vi "DOE Dryer NI Data Compile.vi"(4 "Module Data 6":string[][](array[string]), 5 "Module Data 7":string[][](array[string]), 6 "Module Data 5":string[][](array[string]), 7 "Module Data 1":string[][](array[string]), 8 "Error In":errorcluster, 9 "Module Data 4":string[][](array[string]), 10 "Module Data 3":string[][](array[string]), 11 "Module Data 2":string[][](array[string])) -> (0 "Error Out":errorcluster, 3 "Data Output":string[][](array[string]))   [LabVIEW 2018]
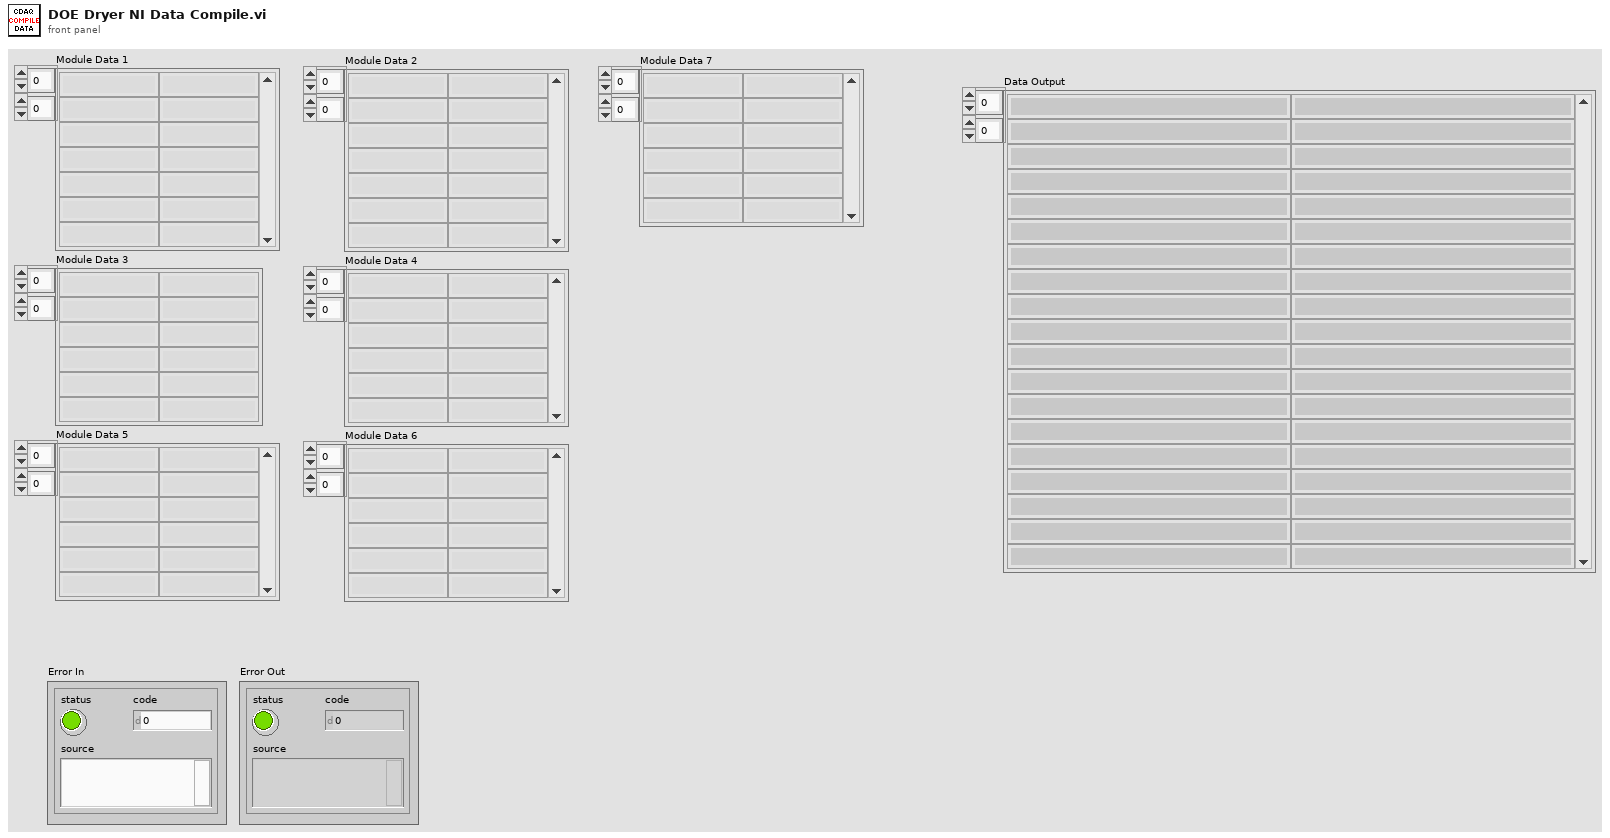
[diagram p1: front panel]
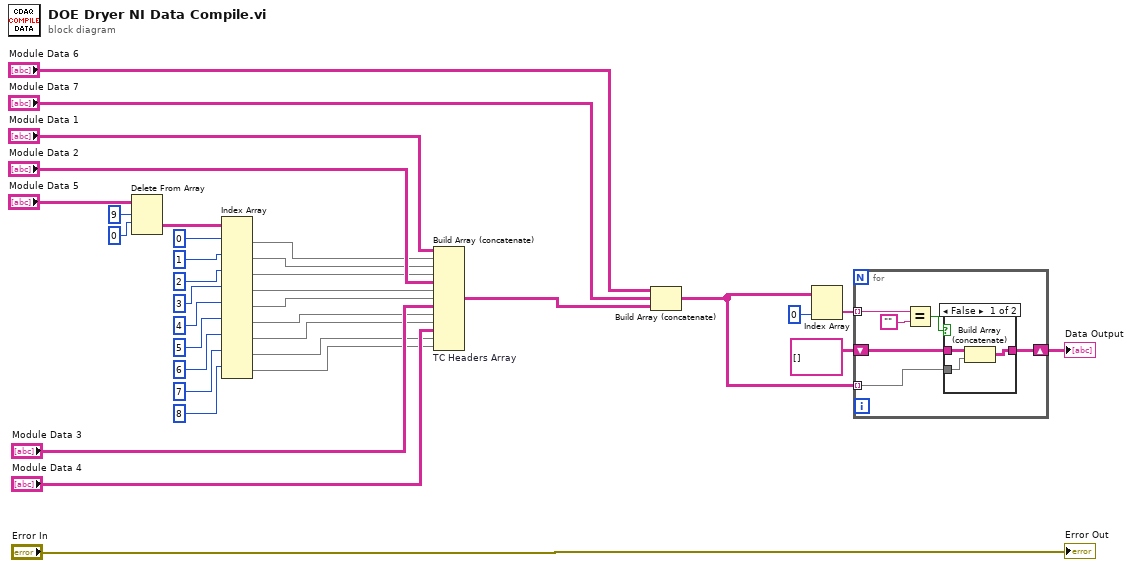
[diagram p0: block diagram]
diagram:
  n1 = Delete From Array(array="Module Data 5", length=9, index (row)=0 ("index")) -> (deleted portion=w30:string[][])  [unwired: 1 in, 1 out]
  n2 = Index Array(array=w30, index (row) #1=0 ("index"), index (row) #2=1 ("index"), index (row) #3=2 ("index"), index (row) #4=3 ("index"), index (row) #5=4 ("index"), index (row) #6=5 ("index"), index (row) #7=6 ("index"), index (row) #8=7 ("index"), index (row) #9=8 ("index")) -> (element #1=w13:string[], element #2=w14:string[], element #3=w15:string[], element #4=w18:string[], element #5=w19:string[], element #6=w22:string[], element #7=w23:string[], element #8=w26:string[], element #9=w27:string[])  [unwired: 9 in]
  n3 = Build Array (concatenate) "TC Headers Array"("Module Data 1", w13, w14, w15, "Module Data 2", w18, w19, "Module Data 3", w22, w23, "Module Data 4", w26, w27) -> (w35:string[][])
  n4 = Build Array (concatenate) ("Environment Data Array")("Module Data 6", "Module Data 7", w35) -> (w4:string[][])
  n5 = Index Array(array=w4, index (col)=0 ("disabled index (col)")) -> (element=w6:string[])  [unwired: 1 in]
  n6 = for {
    tunnel: w6 -> [w41] mode=indexing
    shift-right: [w37] -> w3
    shift-left: string[][] [] -> [w38]
    tunnel: w4 -> [w36] mode=indexing
    n7 = Equal?(x=w41, y="") -> (x = y?=w39:bool)
    n8 = case shown="False" w39 {
      tunnel: w38 -> [w44 w45]
      tunnel: [w43 w45] -> w37
      tunnel: w36 -> [w42 _]
      frame False {
        n9 = Build Array (concatenate)(w44, w42) -> (w43:string[][])
      }
      frame True {
      }
    }
  }
  "Data Output" <- w3
  "Error Out" <- "Error In"
